vi "Initialize Scalar Datatypes and Refs.vi"(8 "error in (no error)":errorcluster, 9 "session in":u32, 10 "Registers":T1[](array[typedef]) {"Register"."Data Type" format="%.0x"}) -> (0 "error out":errorcluster, 2 "Registers Ref":T5[](array[typedef]) {"Data Type" format="%.0x"})   [LabVIEW 2018, in "FPGA Addon Engine.lvlib"]
uses:
  FPGA Addon Engine.lvlib
  Types/Register Settings.ctl
  Addon Shared/Types/Data Type.ctl
  Addon Shared/Types/Scalar Type.ctl
  Addon Shared/Types/Compiled.RegisterSettings.ctl
  Addon Shared/Types/Register Information.ctl
  Addon Shared/FPGA Addon Shared.lvlib
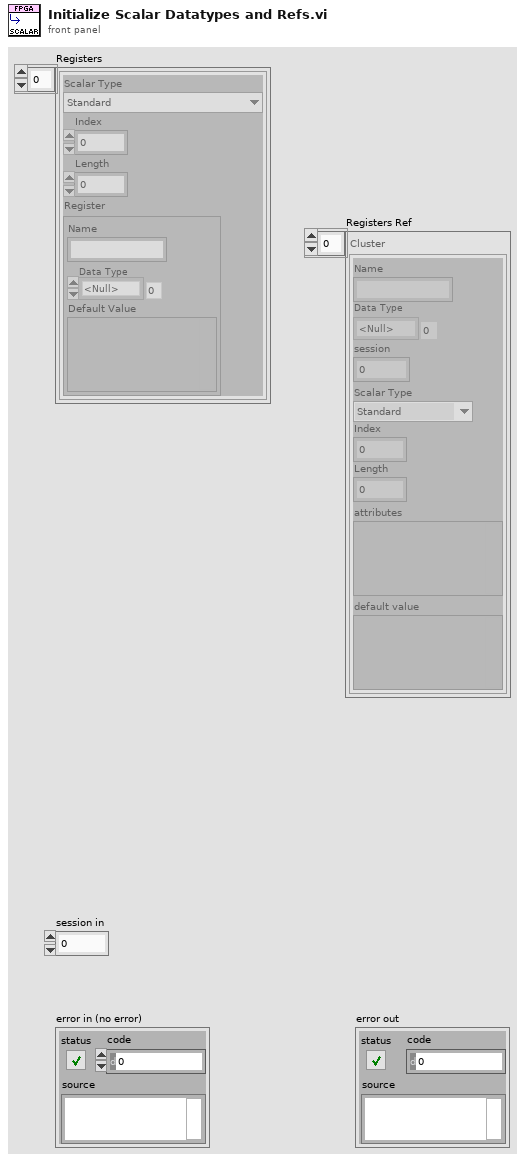
[diagram p1: front panel]
types:
  T1 = typedef "FPGA Addon Shared.lvlib/Compiled.RegisterSettings.ctl" = cluster{"Scalar Type":T2, "Index":i32, "Length":i32, "Register":T3}
  T2 = typedef "FPGA Addon Shared.lvlib/Scalar Type.ctl" = enum16{"Standard", "Bitpacked"}
  T3 = typedef "FPGA Addon Shared.lvlib/Register Information.ctl" = cluster{"Name":string, "Data Type":T4, "Default Value":variant}
  T4 = typedef "FPGA Addon Shared.lvlib/Data Type.ctl" = enum8{"<Null>", "I8", "I16", "I32", "I64", "U8", "U16", "U32", "U64", "SGL", "Boolean", "Analog PWM In Settings", "Analog PWM In", "Digital PWM In Settings", "Digital PWM In", "Digital PWM Out", "Sine Out", "FXP+/-24.5", "FXP+/-16.5", "FXP+/-32.8", "FXP+/-64.32", "FXP+/-16.7", "FXP+/-20.5", "FXP+/-27.5", "FXP+/-32.16", "FXP+16.3", "FXP+18.3", "Digital Static In", "Digital Static Out", "Digital Static In Settings", "Digital WSS Out", "Quad Encoder Settings", "Quad Encoder In", "Group"}
  T5 = typedef "FPGA Addon Engine.lvlib/Register Settings.ctl" = cluster{"Name":string, "Data Type":T4, "session":u32, "Scalar Type":T2, "Index":i32, "Length":i32, "attributes":variant, "default value":variant}
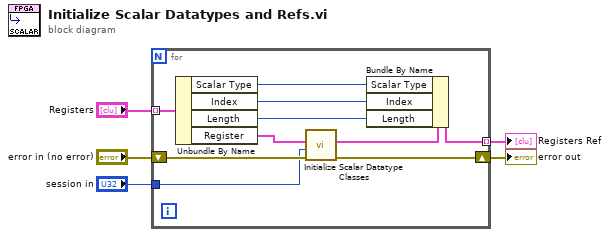
[diagram p0: block diagram]
diagram:
  n1 = for {
    tunnel: [w14] -> w5 mode=indexing
    tunnel: "Registers" -> [w13] mode=indexing
    shift-right: [w7] -> w3
    shift-left: "error in (no error)" -> [w8]
    tunnel: "session in" -> [w6]
    n2 = Unbundle By Name(w13) -> ("Scalar Type"=w9:T2, "Index"=w10:i32, "Length"=w11:i32, "Register"=w12:T3)
    n3 = call "Initialize Scalar Datatype Classes.vi"("error in (no error)"=w8, "session in"=w6, "Register"=w12) -> ("error out"=w7:errorcluster, "Register"=w15:T5)  [unwired: 7 in]
    n4 = Bundle By Name(cluster=w15, "Scalar Type"=w9, "Index"=w10, "Length"=w11) -> (w14:T5)
  }
  "error out" <- w3
  "Registers Ref" <- w5
